vi "纳清DO电极校准.vi"() -> ()   [LabVIEW 2016, in "斯坦道多参数.lvlib"]
uses:
  <vilib>/Utility/miscctls.llb/LVPointTypeDef.ctl
  <vilib>/Analysis/NI_AALBase.lvlib
panel:
  in  "盐度自动获取":bool
  out "滤波设定":dbl
  out "标液2":string="饱和标准液"
  out "标液1":string="零点标准液"
  out "第二点信号值":dbl
  out "第一点信号值":dbl
  out "盐度":sgl format="%#.2f"
  out "大气压力":dbl format="%#.2f"
  out "饱和值":sgl format="%#.2f"
  out "报警信息":string
  out "通讯状态":string
  out "第二点校准值":dbl
  out "第一点校准值":dbl
  in  "校准停止":bool
  in  "校准启动":bool
  in  "校准模式":u16(ring)=1 items=["两点校准", "单点校准"]
  out "最小值":sgl format="%#.2f"
  out "最大值":sgl format="%#.2f"
  out "波形图表":dbl(graph) caption="历史曲线"
  out "mean":dbl caption="均值" format="%#.2f"
  out "standard deviation":dbl caption="标准差" format="%#.2f"
  out "变异系数":dbl format="%#.6f"
  out "测量值":sgl format="%#.2f"
  out "提示":string
  out "原始光强数值":sgl caption="信号值" format="%#.6f"
  out "温度":dbl format="%#.2f"
  # "DO电极设定"
  # "℃"
  # "mg/L"
  # "%"
  # "nA"
  # "kPa"
  # "ppt"
  # "请选择校准模式:"
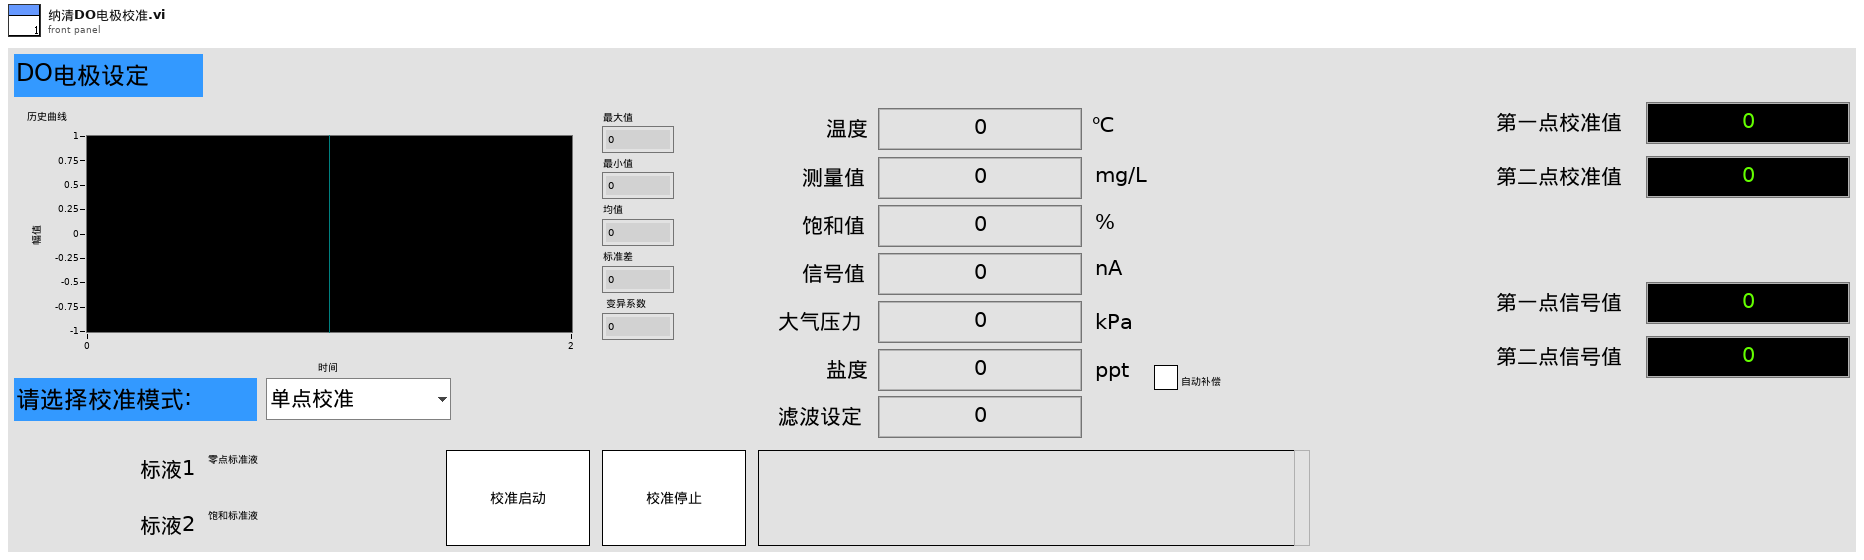
[diagram p1: front panel]
types:
  T1 = enum16{"pH", "DO", "Cond", "Turb", "ORP", "叶绿素a", "藻密度"}
  T2 = typedef "LVPointTypeDef.ctl" = cluster{"Horizontal":i16, "Vertical":i16}
  T3 = cluster{"报警码":u16, "溶解氧数值（mg/L）":sgl, "溶解氧数据（%）":sgl, "温度数据":sgl, "溶解氧原始信号 nA":sgl, "大气压力":sgl, "盐度":sgl, "0X0009_NC":string, "产品名称":string, "序列号":string, "硬件版本":string, "软件版本":string, "通讯地址":u16, "波特率":u16, "设备类型":u16, "0X0026_NC":string, "第一点原始数据":sgl, "第一点校准数据":sgl, "第二点原始数据":sgl, "第二点校准数据":sgl, "探头校准命令":u16, "温度校准参数":sgl, "温度校准命令":u16}
  T4 = cluster{"pH":u32, "DO":u32, "Cond":u32, "Turb":u32, "叶绿素a":u32, "藻密度":u32, "ORP":u32}
  T5 = enum8{"Enabled", "Disabled", "Disabled and Grayed Out"}
  T6 = cluster{"报警码":u16, "溶解氧数值（mg/L）":sgl, "溶解氧数据（%）":sgl, "温度数据":sgl, "溶解氧原始信号 nA":sgl, "大气压力":sgl, "盐度":sgl, "0X0009_NC":string, "产品名称":string, "序列号":string, "硬件版本":string, "软件版本":string, "通讯地址":u16, "波特率":u16, "设备类型":u16, "0X0026_NC":string, "第一点原始数据":sgl, "0X0033 NC":sgl, "第二点原始数据":sgl, "0X0037 NC":sgl, "探头校准命令":u16, "温度校准参数":sgl, "温度校准命令":u16}
  T7 = cluster{"ph":bool, "DO":bool, "Cond":bool, "Turb":bool, "叶绿素a":bool, "藻密度":bool, "ORP":bool}
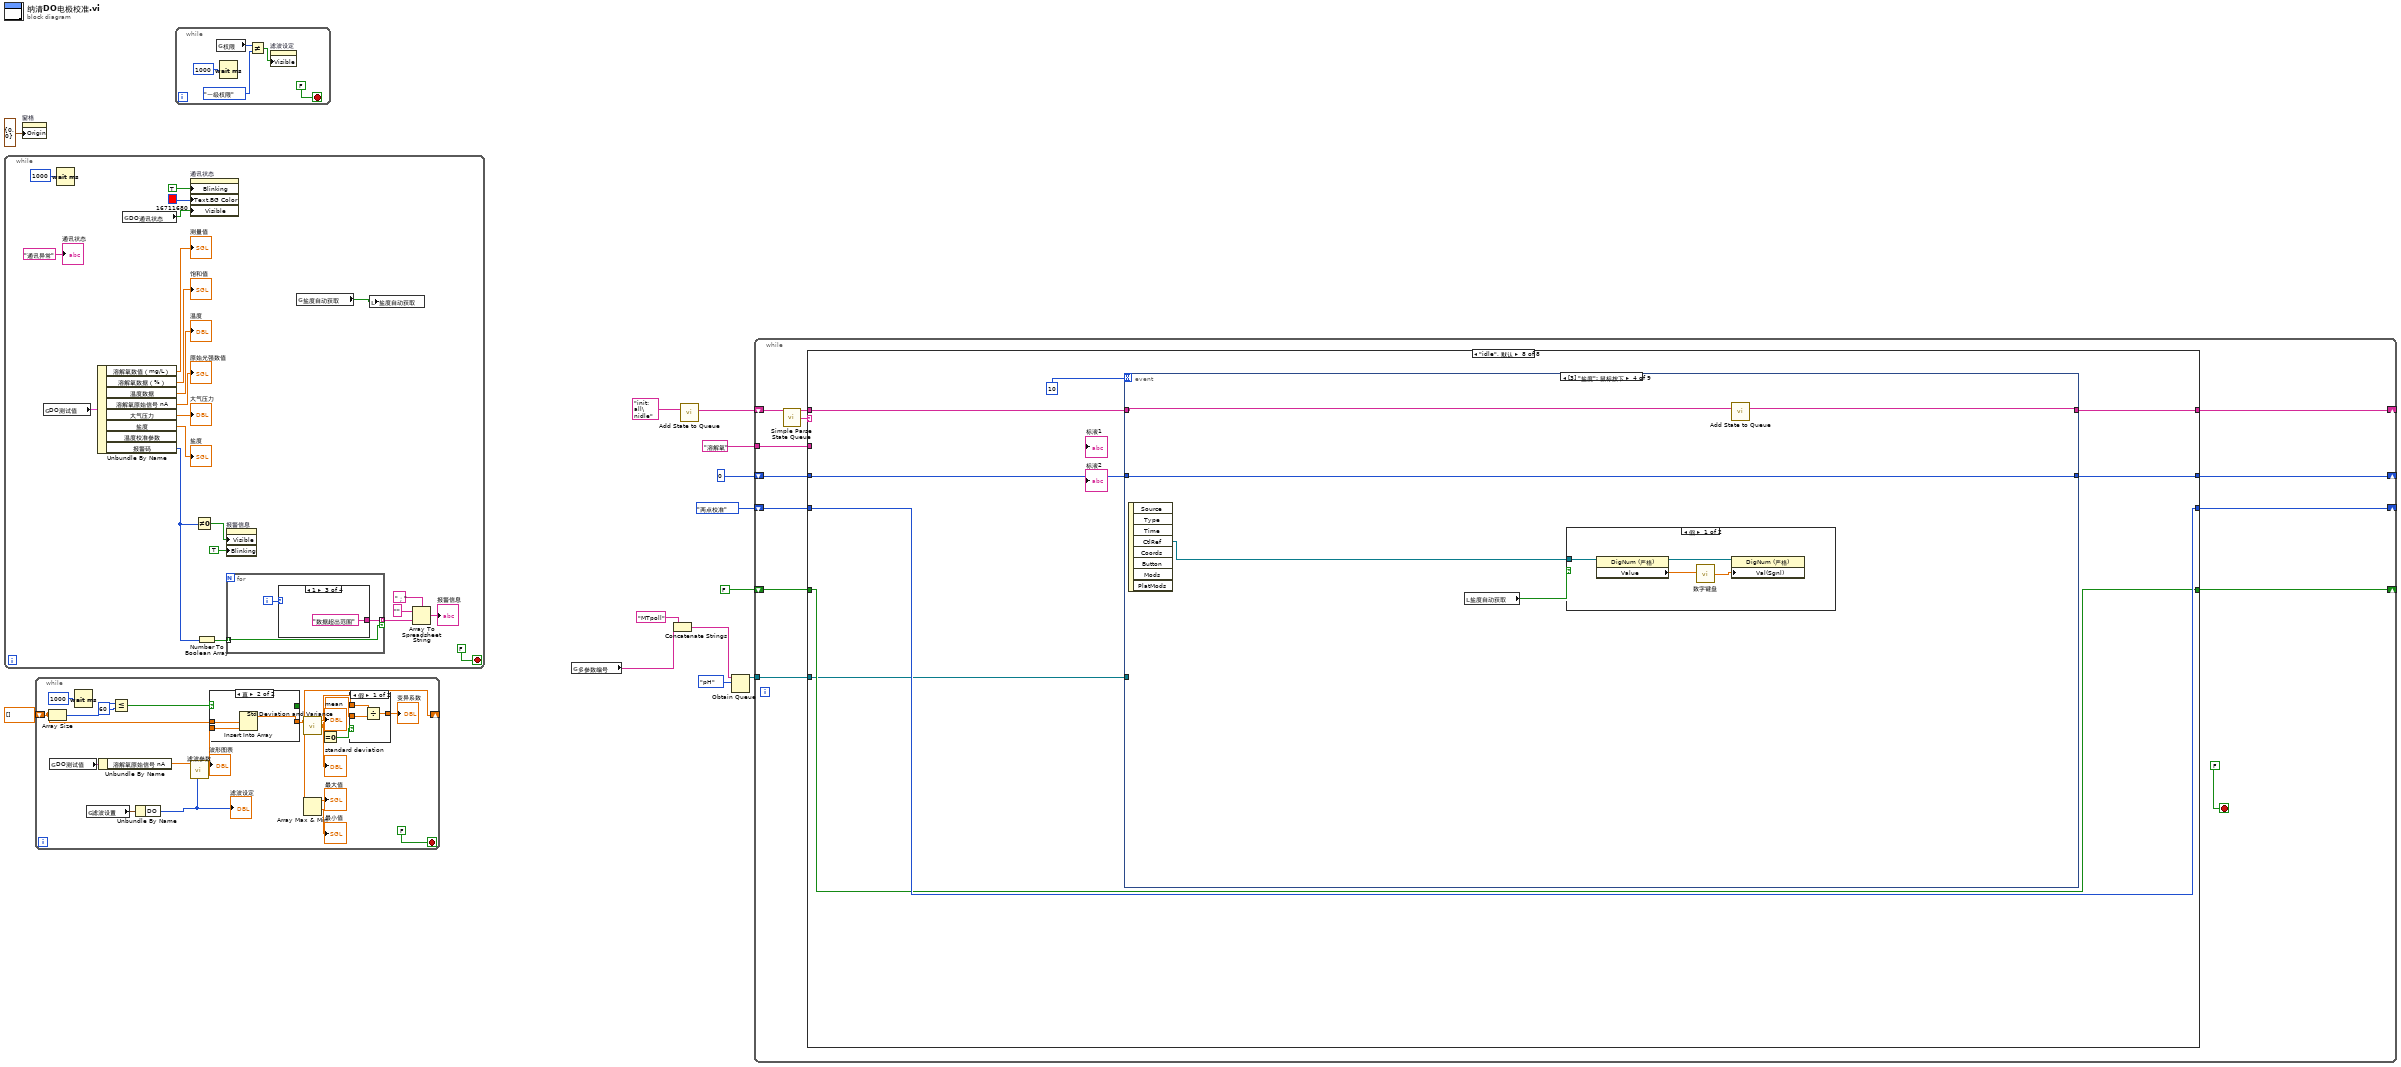
[diagram p0: block diagram]
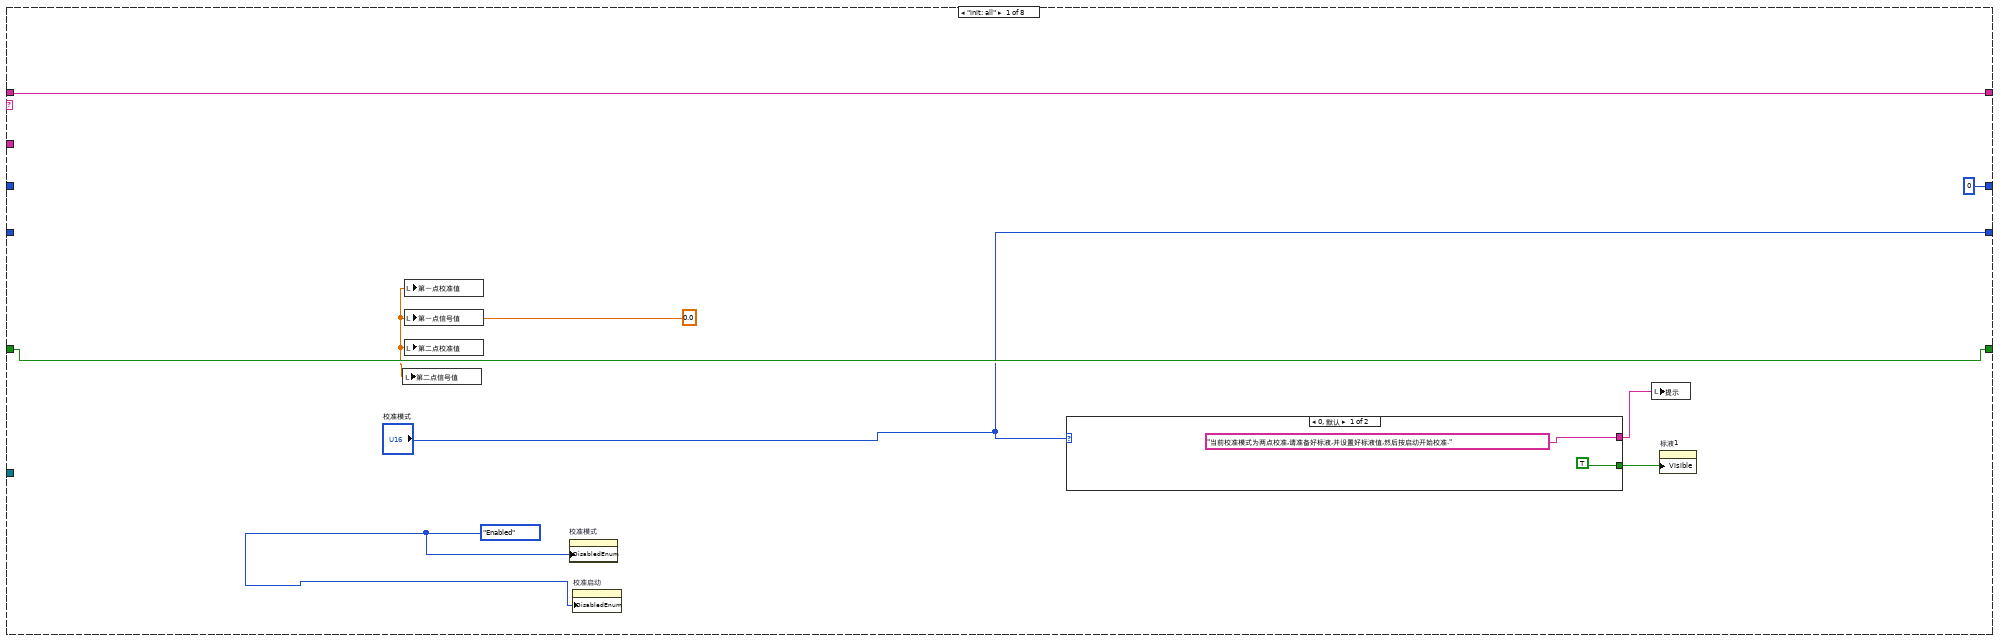
[diagram p2: hidden frame]
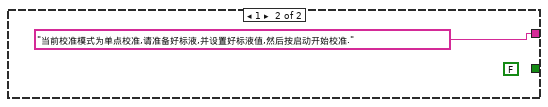
[diagram p3: hidden frame]
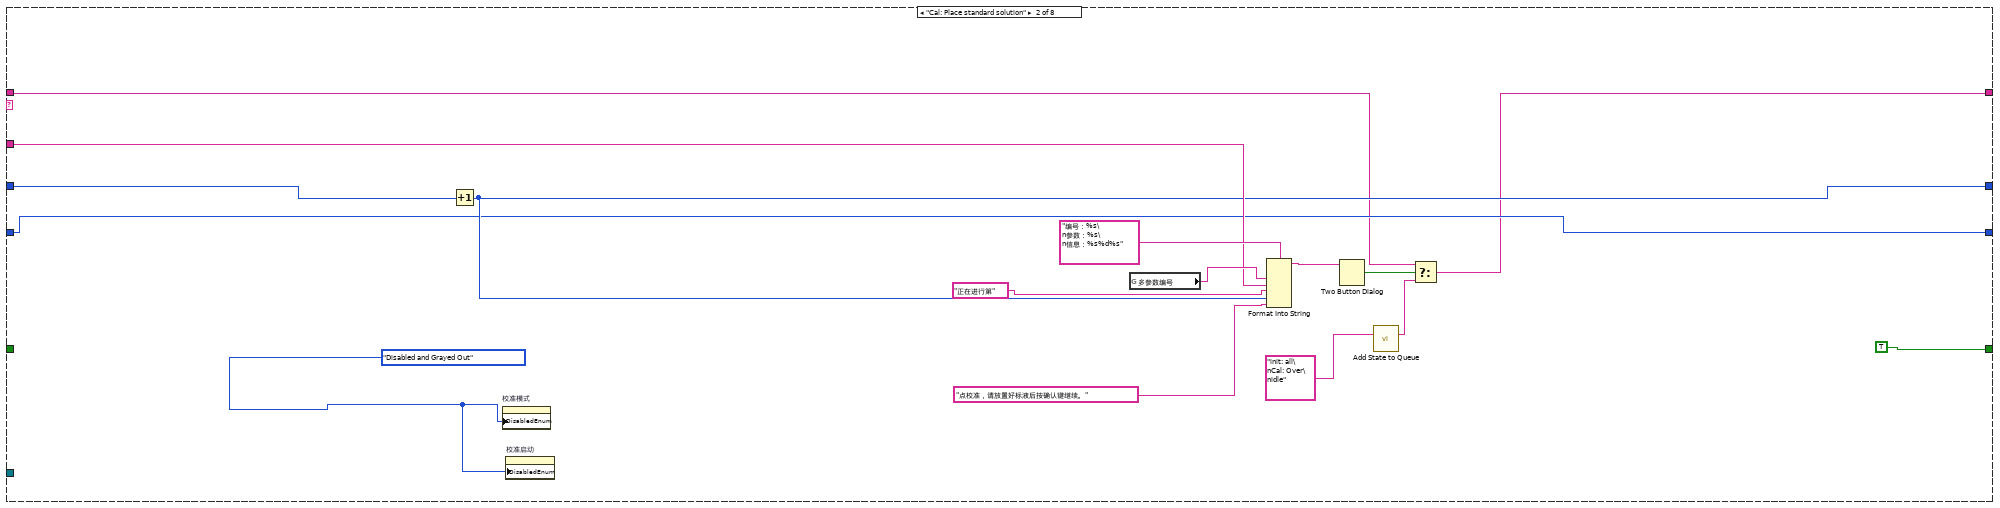
[diagram p4: hidden frame]
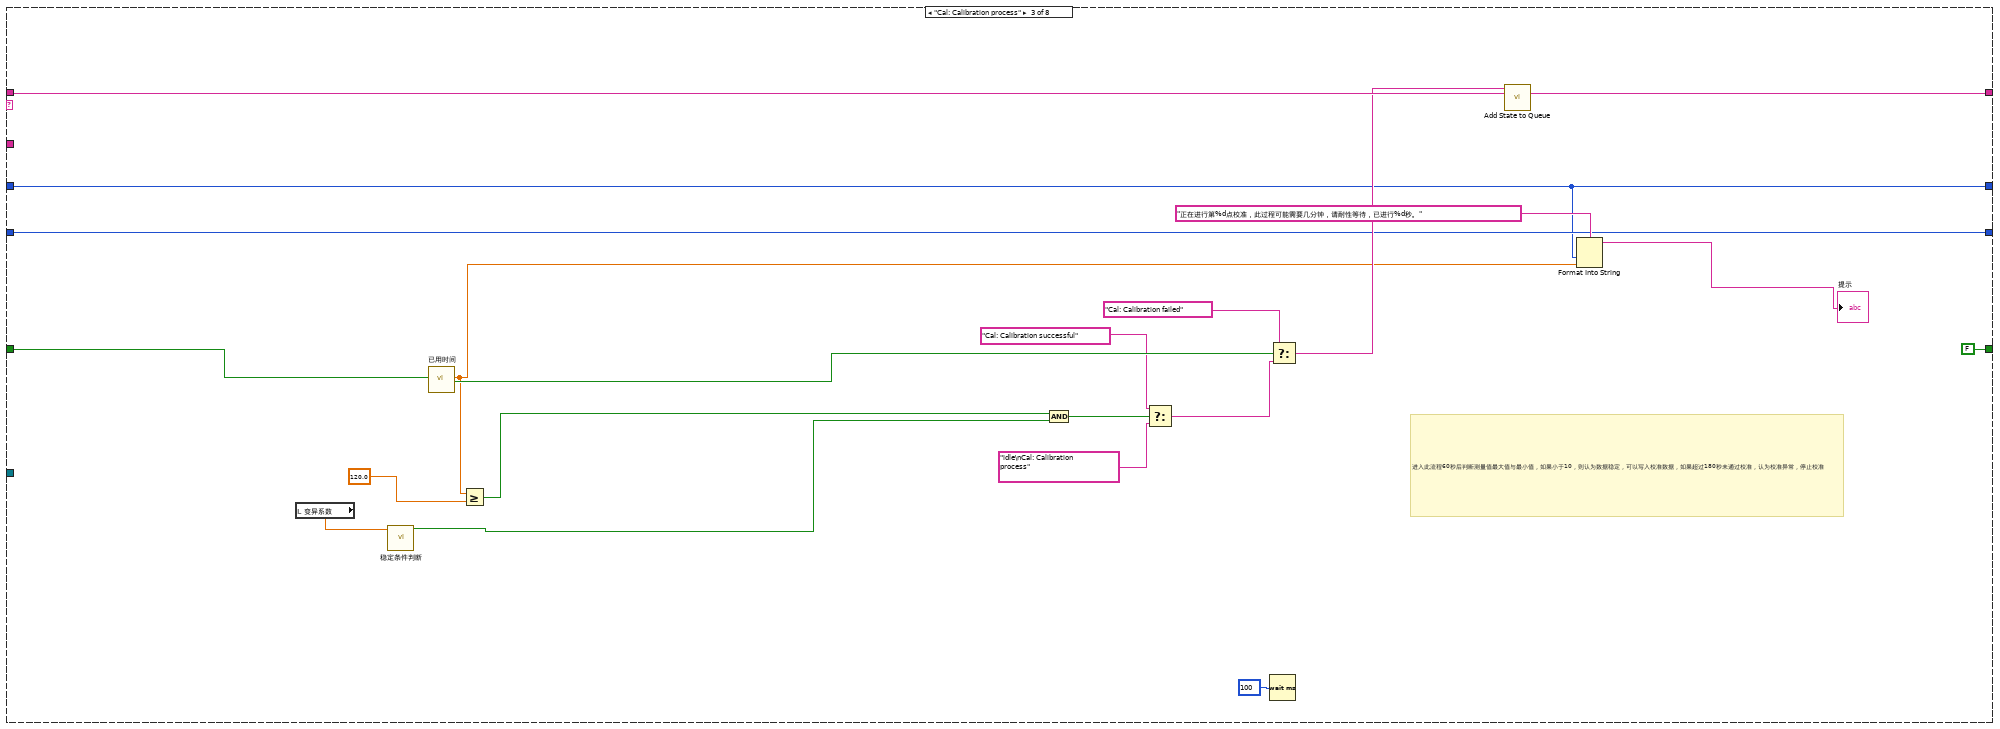
[diagram p5: hidden frame]
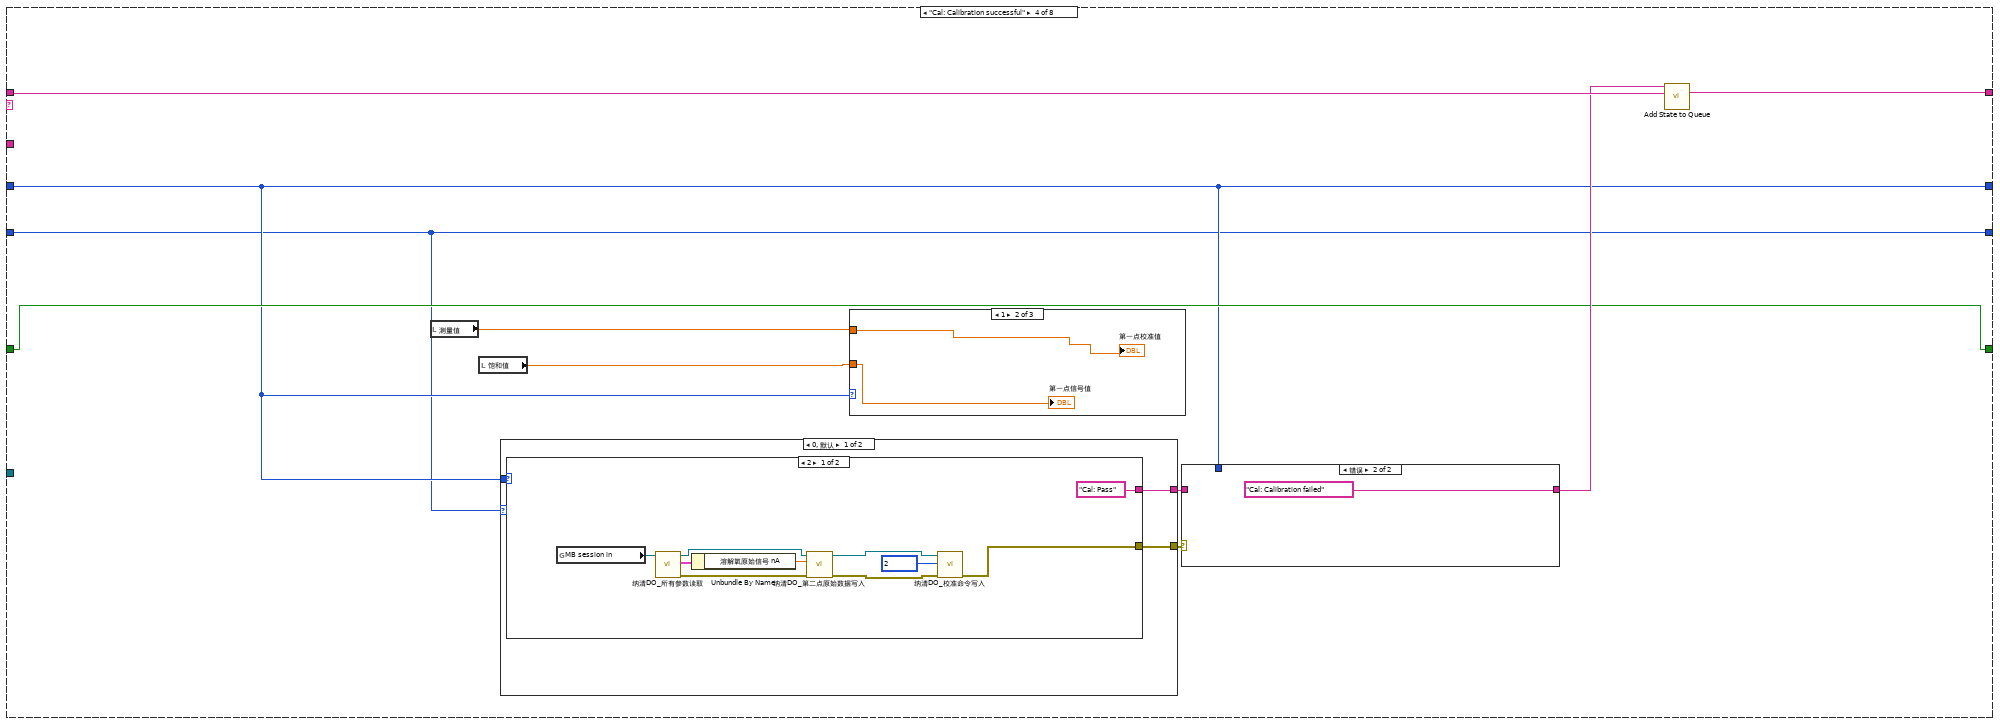
[diagram p6: hidden frame]
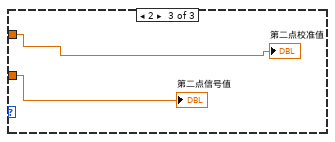
[diagram p8: hidden frame]
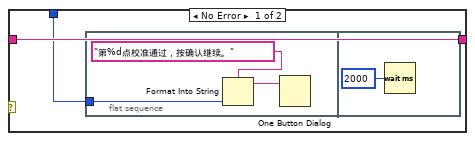
[diagram p9: hidden frame]
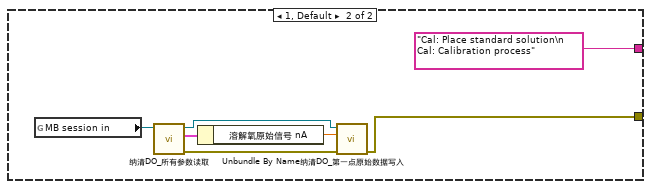
[diagram p10: hidden frame]
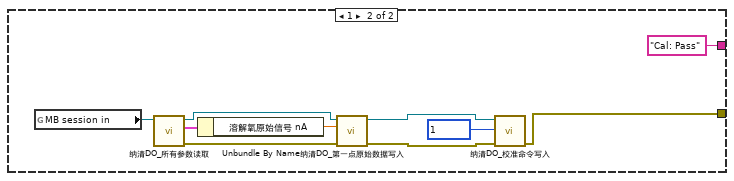
[diagram p11: hidden frame]
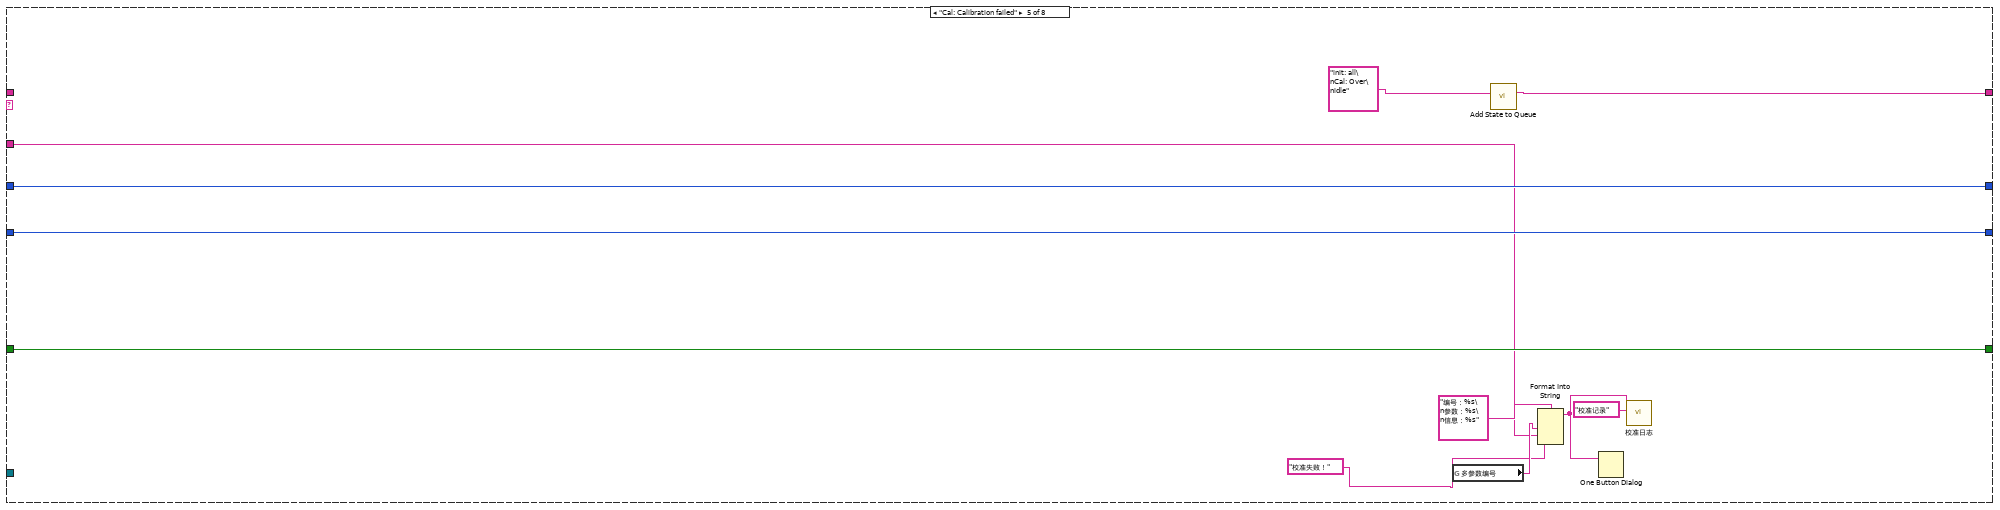
[diagram p12: hidden frame]
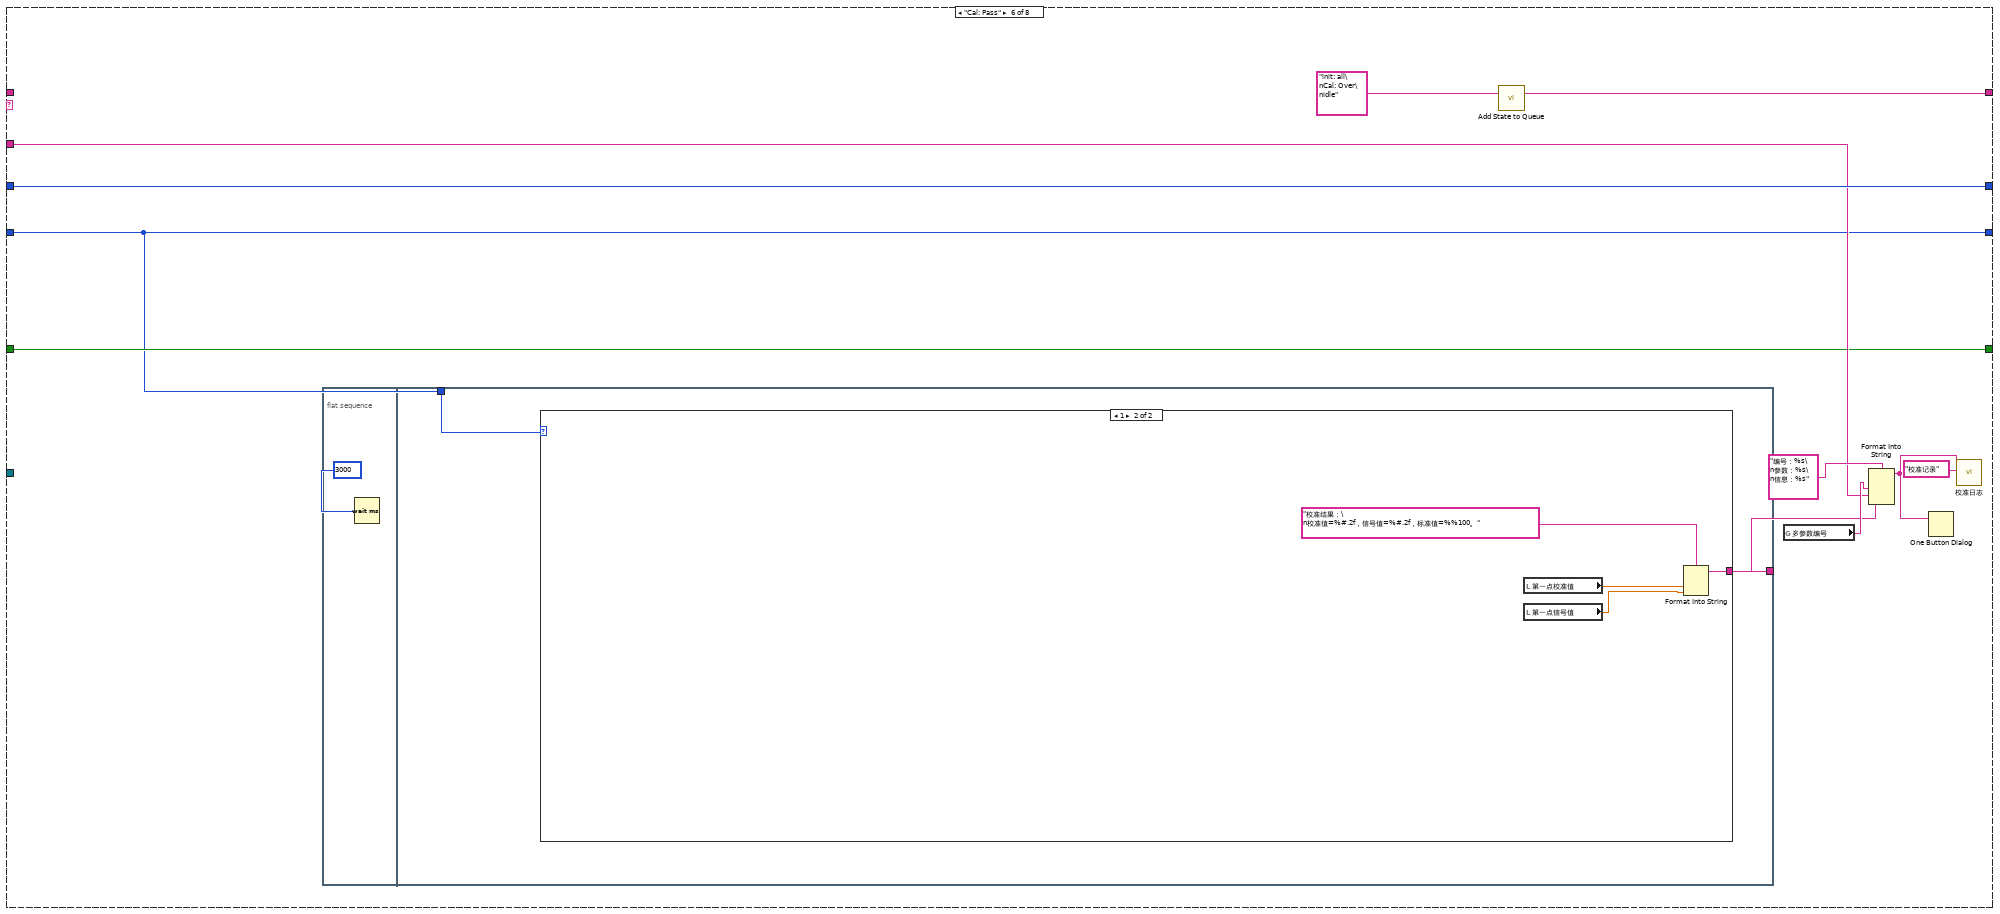
[diagram p13: hidden frame]
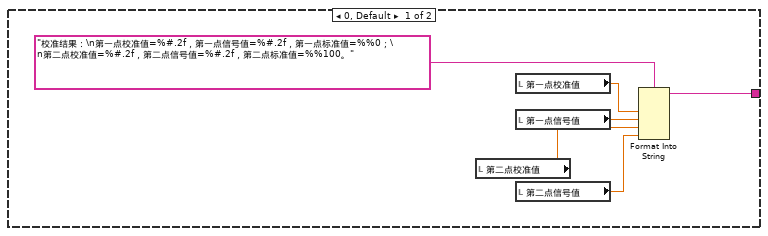
[diagram p14: hidden frame]
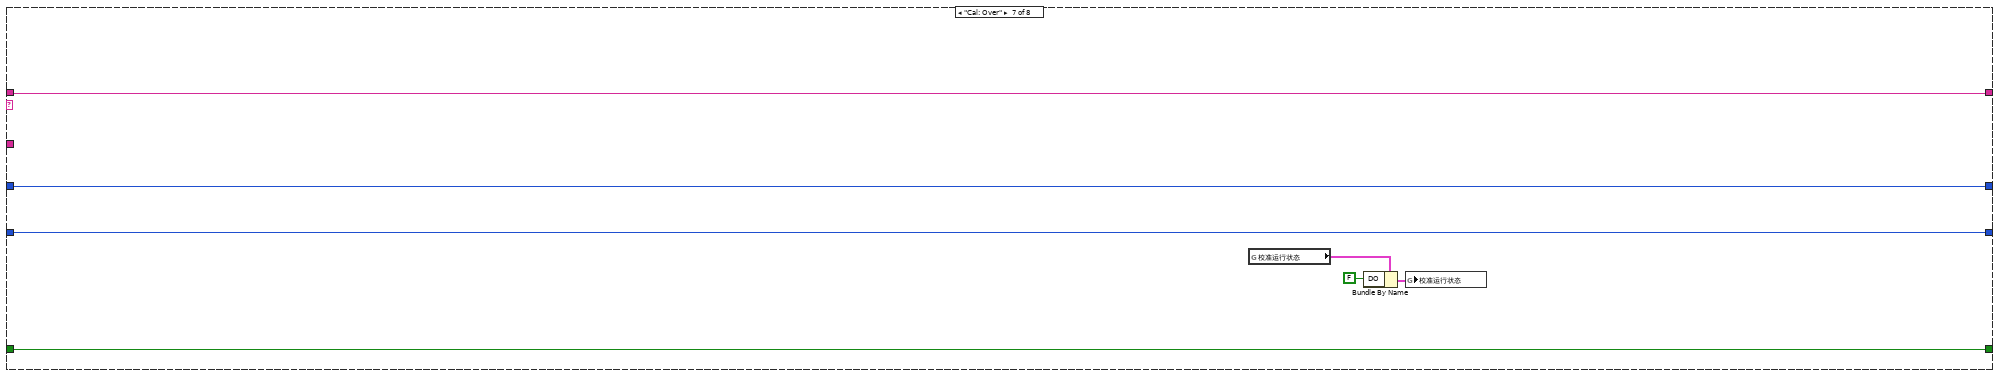
[diagram p15: hidden frame]
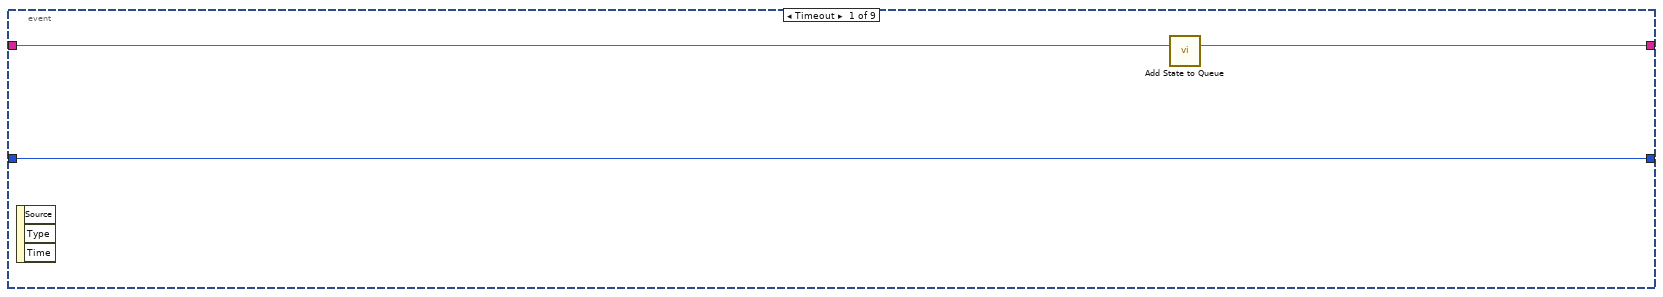
[diagram p16: hidden frame]
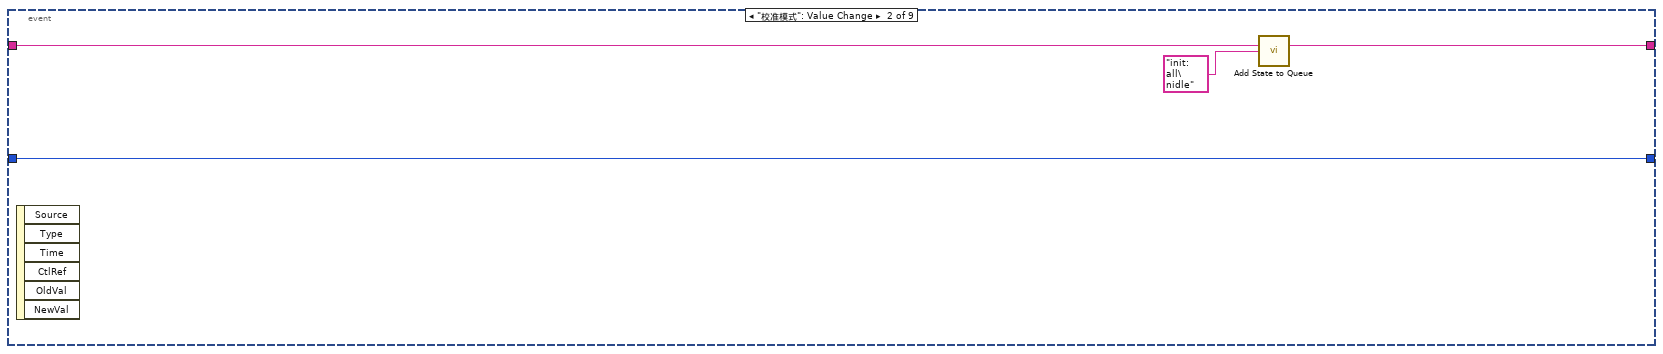
[diagram p17: hidden frame]
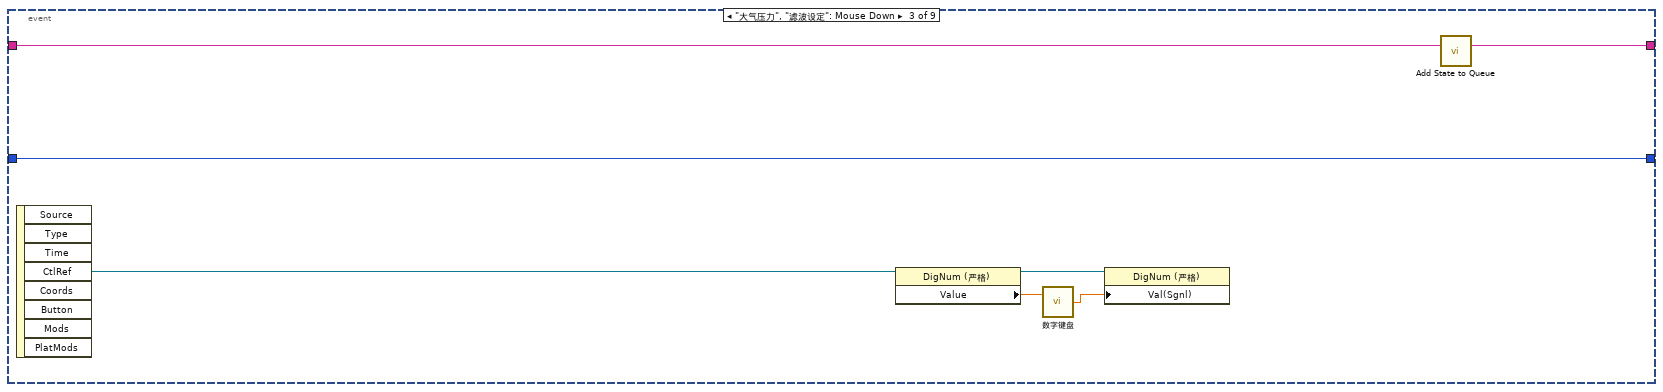
[diagram p18: hidden frame]
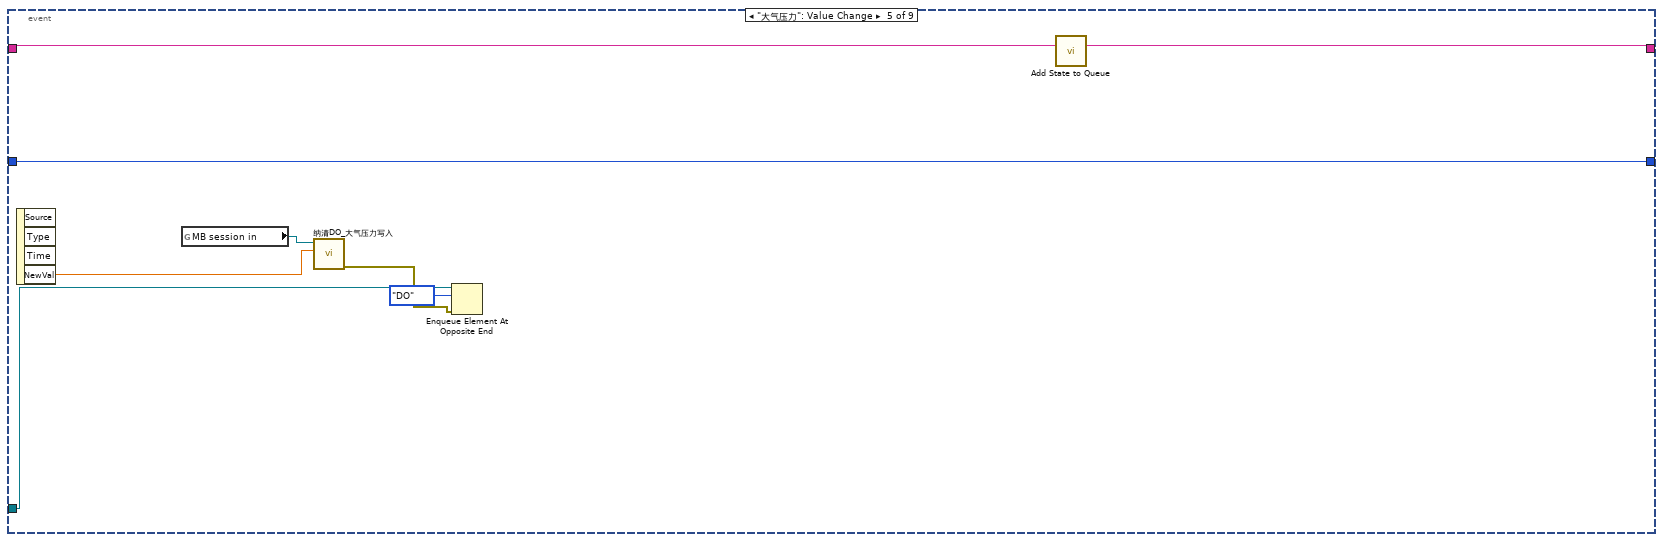
[diagram p20: hidden frame]
diagram:
  n1 = while {
    stop <- FALSE stop-if-true
    n2 = global read "纳清过程全局变量.vi" "DO测试值"() -> (w33:T3)
    n3 = Wait (ms)(milliseconds to wait=u32 1000 ("等待时间（毫秒）")) -> ()  [unwired: 1 out]
    n4 = Unbundle By Name(w33) -> ("溶解氧数值（mg/L）"=→"测量值":sgl, "溶解氧数据（%）"=→"饱和值":sgl, "温度数据"=→"温度":sgl, "溶解氧原始信号 nA"=→"原始光强数值":sgl, "大气压力"=→"大气压力":sgl, "盐度"=→"盐度":sgl, "报警码"=w20:u16)  [unwired: 1 out]
    n5 = global read "多参数全局变量.vi" "DO通讯状态"() -> (w26:bool)
    n6 = property on="通讯状态" class="Str"("Blinking"=TRUE ("闪烁"), "Text.BG Color"=u32 16711680, "Visible"=w26) -> ()  [unwired: 2 in, 2 out]
    n7 = Not Equal To 0?(x=w20) -> (x != 0?=w19:bool)
    n8 = Number To Boolean Array(number=w20) -> (Boolean array=w25:bool[])
    n9 = property on="报警信息" class="Str"("Visible"=w19, "Blinking"=TRUE ("闪烁")) -> ()  [unwired: 2 in, 2 out]
    n10 = for {
      tunnel: w25 -> [w36] mode=indexing
      tunnel: [w37] -> w24 mode=indexing if=w36
      i -> [w38]
      n11 = case shown="1" w38 {
        tunnel: [_ "温度超出范围" "数据超出范围" "温度传感器故障"] -> w37
        frame Default {
        }
        frame 0 {
        }
        frame 1 {
        }
        frame 8 {
        }
      }
    }
    n12 = global read "断电保存变量.vi" "盐度自动获取"() -> (w14:bool)
    n13 = local write "盐度自动获取"(w14) -> ()
    n14 = Array To Spreadsheet String(delimiter (Tab)="；" ("分隔符(Tab)"), array=w24, 3:"" ("格式字符串")) -> (spreadsheet string=→"报警信息":string)
    "通讯状态" <- "通讯异常" ("当前串口")
  }
  n15 = property on="窗格" class="Pane"("Origin"=T2 {"Horizontal"=0, "Vertical"=0} ("原点")) -> ()  [unwired: 2 in, 2 out]
  n16 = while {
    shift-right: [w49] -> _
    shift-left: sgl[] [] -> [w55]
    stop <- FALSE stop-if-true
    n17 = Array Size(array=w55) -> (size(s)=w57:i32)
    n18 = global read "纳清过程全局变量.vi" "DO测试值"() -> (w46:T3)
    n19 = Wait (ms)(milliseconds to wait=u32 1000 ("等待时间（毫秒）")) -> ()  [unwired: 1 out]
    n20 = global read "断电保存变量.vi" "滤波设置"() -> (w43:T4)
    n21 = Unbundle By Name(w46) -> ("溶解氧原始信号 nA"=w45:sgl)
    n22 = Less Or Equal?(x=w57, y=60) -> (x <= y?=w56:bool)
    n23 = Unbundle By Name(w43) -> ("DO"=w42:u32)
    "滤波设定" <- w42
    n24 = call "滤波参数.vi"("滤波次数"=w42, "x"=w45) -> ("mode"=w44:dbl)  [unwired: 9 in]
    "波形图表" <- w44
    n25 = case shown="真" w56 {
      tunnel: w55 -> [w68 w71]
      tunnel: w44 -> [w66 w70]
      tunnel: [w64 w69] -> w49
      tunnel: [TRUE _] -> _
      frame False {
        n26 = Replace Array Subset(array=w68, new element=w66) -> (w67:sgl[])  [unwired: 1 in]
        n27 = Rotate 1D Array(1:w67, 2:-1 ("n")) -> (0:w64:sgl[])
      }
      frame True {
        n28 = Insert Into Array(array=w71, new element=w70) -> (w69:sgl[])  [unwired: 1 in]
      }
    }
    n29 = call <vilib>:"Std Deviation and Variance.vi"("X"=w49) -> ("mean"=w53:dbl, "standard deviation"=w52:dbl)  [unwired: 1 in, 1 out]
    "mean" <- w53
    "standard deviation" <- w52
    n30 = Array Max & Min(array=w49) -> (max value=→"最大值":sgl, min value=→"最小值":sgl)  [unwired: 2 out]
    n31 = Equal To 0?(x=w53) -> (x = 0?=w54:bool)
    n32 = case shown="假" w54 {
      tunnel: w52 -> [w62 _]
      tunnel: [w61 _] -> w51
      tunnel: w53 -> [w60 _]
      frame False {
        n33 = Divide(x=w62, y=w60) -> (x/y=w61:dbl)
      }
      frame True {
      }
    }
    "变异系数" <- w51
  }
  n34 = while {
    stop <- FALSE stop-if-true
    n35 = global read "多参数全局变量.vi" "权限"() -> (w75:enum16{"一级权限", "二级权限", "三级权限"})
    n36 = Wait (ms)(milliseconds to wait=u32 1000 ("等待时间（毫秒）")) -> ()  [unwired: 1 out]
    n37 = Not Equal?(x=w75, y=enum16{"一级权限", "二级权限", "三级权限"}."一级权限") -> (x != y?=w72:bool)
    n38 = property on="滤波设定" class="DigNum (严格)"("Visible"=w72) -> ()  [unwired: 2 in, 2 out]
  }
  n39 = global read "多参数全局变量.vi" "多参数编号"() -> (w2:string)
  n40 = Concatenate Strings("MTpoll" ("名称（未命名）"), w2) -> (w4:string)
  n41 = call "Add State to Queue.vi"("State(s) In (\"\")"="init: all\nidle" ("State(s) In (\"\")")) -> ("States Out"=w10:string)  [unwired: 14 in]
  n42 = Obtain Queue(name (unnamed)=w4, element data type=T1."pH" ("枚举")) -> (queue out=w1:refnum<queue>)  [unwired: 3 in, 2 out]
  n43 = while {
    shift-right: [w85] -> _
    shift-left: w10 -> [w89]
    shift-right: [w82] -> _
    shift-left: 0 -> [w84]
    tunnel: "溶解氧" ("State(s) In (\"\")") -> [w83]
    shift-right: [w80] -> _
    shift-left: enum16{"两点校准", "单点校准"}."两点校准" ("校准模式") -> [w81]
    shift-right: [w78] -> _
    shift-left: FALSE -> [w79]
    tunnel: w1 -> [w77]
    stop <- FALSE stop-if-true
    n44 = call "Simple Parse State Queue.vi"("State Queue"=w89) -> ("Remain States"=w86:string, "Next State"=w87:string)  [unwired: 13 in]
    n45 = case shown="\"idle\", 默认" w87 {
      tunnel: w86 -> [w97 w104 w136 w145 _ _ w230 w238]
      tunnel: [w97 w103 w135 w144 w196 w201 w230 w237] -> w85
      tunnel: w84 -> [_ w112 w121 w139 w199 w210 w229 w235]
      tunnel: w83 -> [_ w113 _ _ w190 w206 _ _]
      tunnel: [0 w110 w121 w139 w199 w210 w229 w236] -> w82
      tunnel: w81 -> [_ w109 w122 w138 w198 w202 w228 w234]
      tunnel: ["校准模式" w109 w122 w138 w198 w202 w228 w234] -> w80
      tunnel: w79 -> [w94 _ w124 w140 w197 w205 w227 w232]
      tunnel: [w94 TRUE FALSE w140 w197 w205 w227 w232] -> w78
      tunnel: w77 -> [_ _ _ _ _ _ _ w231]
      frame "init: all" {
        w91 = T5."Enabled" ("禁用")
        w93 = 0.0 ("第一点校准值")
        n46 = local write "第二点信号值"(w93) -> ()
        n47 = local write "第一点校准值"(w93) -> ()
        n48 = local write "第一点信号值"(w93) -> ()
        n49 = local write "第二点校准值"(w93) -> ()
        n50 = property on="校准模式" class="Ring (严格)"("DisabledEnum"=w91) -> ()  [unwired: 2 in, 2 out]
        n51 = property on="校准启动" class="Bool"("DisabledEnum"=w91) -> ()  [unwired: 2 in, 2 out]
        n52 = case shown="0, 默认" "校准模式" {
          tunnel: ["当前校准模式为两点校准,请准备好标液,并设置好标液值,然后按启动开始校准." ("提示") "当前校准模式为单点校准,请准备好标液,并设置好标液值,然后按启动开始校准." ("提示")] -> w96
          tunnel: [TRUE ("可见") _] -> w90
          frame 0, Default {
          }
          frame 1 {
            (unwired) FALSE ("可见")
          }
        }
        n53 = local write "提示"(w96) -> ()
        n54 = property on="标液1" class="Str"("Visible"=w90) -> ()  [unwired: 2 in, 2 out]
      }
      frame "Cal: Place standard solution" {
        w102 = T5."Disabled and Grayed Out" ("禁用")
        n55 = Increment(x=w112) -> (x+1=w110:i32)
        n56 = property on="校准模式" class="Ring (严格)"("DisabledEnum"=w102) -> ()  [unwired: 2 in, 2 out]
        n57 = property on="校准启动" class="Bool"("DisabledEnum"=w102) -> ()  [unwired: 2 in, 2 out]
        n58 = global read "多参数全局变量.vi" "多参数编号"() -> (w115:string)
        n59 = Format Into String(format string="编号：%s\n参数：%s\n信息：%s%d%s" ("格式字符串"), w115, w113, "正在进行第" ("消息"), w110, "点校准，请放置好标液后按确认键继续。" ("消息")) -> (resulting string=w107:string)  [unwired: 2 in, 1 out]
        n60 = Two Button Dialog(message=w107) -> (T button?=w106:bool)  [unwired: 2 in]
        n61 = call "Add State to Queue.vi"("State(s) In (\"\")"="init: all\nCal: Over\nidle" ("State(s) In (\"\")")) -> ("States Out"=w105:string)  [unwired: 14 in]
        n62 = Select(t=w104, s=w106, f=w105) -> (s? t:f=w103:string)
      }
      frame "Cal: Calibration process" {
        # "进入此流程60秒后判断测量值最大值与最小值，如果小于10，则认为数据稳定，可以写入校准数据，如果超过180秒未通过校准，认为校准异常，停止校准"
        n63 = local read "变异系数"() -> (w118:dbl)
        n64 = call "稳定条件判断.vi"("变异系数"=w118) -> ("布尔"=w117:bool)  [unwired: 10 in]
        n65 = call "已用时间"("Reset"=w124) -> ("Elapsed Time (s)"=w120:dbl, "Time has Elapsed"=w137:bool)  [unwired: 11 in, 6 out]
        n66 = Greater Or Equal?(x=w120, y=120.0) -> (x >= y?=w132:bool)
        n67 = And(x=w132, y=w117) -> (x .and. y?=w129:bool)
        n68 = Select(t="Cal: Calibration successful" ("State(s) In (\"\")"), s=w129, f="idle\nCal: Calibration process" ("State(s) In (\"\")")) -> (s? t:f=w128:string)
        n69 = Wait (ms)(milliseconds to wait=u32 100 ("等待时间（毫秒）")) -> ()  [unwired: 1 out]
        n70 = Select(t="Cal: Calibration failed" ("State(s) In (\"\")"), s=w137, f=w128) -> (s? t:f=w127:string)
        n71 = call "Add State to Queue.vi"("State(s) In Front (\"\")"=w127, "State(s) In (\"\")"=w136) -> ("States Out"=w135:string)  [unwired: 13 in]
        n72 = Format Into String(format string="正在进行第%d点校准，此过程可能需要几分钟，请耐性等待，已进行%d秒。" ("格式字符串"), w121, w120) -> (resulting string=→"提示":string)  [unwired: 2 in, 1 out]
      }
      frame "Cal: Calibration successful" {
        n73 = local read "测量值"() -> (w141:sgl)
        n74 = local read "饱和值"() -> (w142:sgl)
        n75 = case shown="0, 默认" w138 {
          tunnel: [w161 w179] -> w147
          tunnel: [w160 "Cal: Pass" ("State(s) In (\"\")")] -> w146
          tunnel: w139 -> [w159 _]
          frame 0, Default {
            n76 = case shown="2" w159 {
              tunnel: [w163 w172] -> w161
              tunnel: ["Cal: Pass" ("State(s) In (\"\")") "Cal: Place standard solution\n Cal: Calibration process" ("State(s) In (\"\")")] -> w160
              frame 2 {
                n77 = global read "多参数全局变量.vi" "MB session in"() -> (w168:refnum<class "MB_Master.lvclass">)
                n78 = call "纳清DO_所有参数读取.vi"("MB session in"=w168) -> ("error out"=w170:errorcluster, "输出值"=w167:T6, "MB session out"=w169:refnum<class "MB_Master.lvclass">)  [unwired: 8 in]
                n79 = Unbundle By Name(w167) -> ("溶解氧原始信号 nA"=w166:sgl)
                n80 = call "纳清DO_第二点原始数据写入.vi"("error in (no error)"=w170, "数值"=w166, "MB session in"=w169) -> ("error out"=w165:errorcluster, "MB session out"=w164:refnum<class "MB_Master.lvclass">)  [unwired: 7 in]
                n81 = call "纳清DO_校准命令写入.vi"("error in (no error)"=w165, "数值"=u16 2 ("starting address"), "MB session in"=w164) -> ("error out"=w163:errorcluster)  [unwired: 7 in, 1 out]
              }
              frame 1, Default {
                n82 = global read "多参数全局变量.vi" "MB session in"() -> (w175:refnum<class "MB_Master.lvclass">)
                n83 = call "纳清DO_所有参数读取.vi"("MB session in"=w175) -> ("error out"=w177:errorcluster, "输出值"=w174:T6, "MB session out"=w176:refnum<class "MB_Master.lvclass">)  [unwired: 8 in]
                n84 = Unbundle By Name(w174) -> ("溶解氧原始信号 nA"=w173:sgl)
                n85 = call "纳清DO_第一点原始数据写入.vi"("error in (no error)"=w177, "数值"=w173, "MB session in"=w176) -> ("error out"=w172:errorcluster)  [unwired: 7 in, 1 out]
              }
            }
          }
          frame 1 {
            n86 = global read "多参数全局变量.vi" "MB session in"() -> (w185:refnum<class "MB_Master.lvclass">)
            n87 = call "纳清DO_所有参数读取.vi"("MB session in"=w185) -> ("error out"=w187:errorcluster, "输出值"=w184:T6, "MB session out"=w186:refnum<class "MB_Master.lvclass">)  [unwired: 8 in]
            n88 = Unbundle By Name(w184) -> ("溶解氧原始信号 nA"=w183:sgl)
            n89 = call "纳清DO_第一点原始数据写入.vi"("error in (no error)"=w187, "数值"=w183, "MB session in"=w186) -> ("error out"=w182:errorcluster, "MB session out"=w181:refnum<class "MB_Master.lvclass">)  [unwired: 7 in]
            n90 = call "纳清DO_校准命令写入.vi"("error in (no error)"=w182, "数值"=u16 1 ("starting address"), "MB session in"=w181) -> ("error out"=w179:errorcluster)  [unwired: 7 in, 1 out]
          }
        }
        n91 = case shown="1" w139 {
          tunnel: w142 -> [_ w149 w151]
          tunnel: w141 -> [_ w148 w150]
          frame 0, Default {
          }
          frame 1 {
            "第一点信号值" <- w149
            "第一点校准值" <- w148
          }
          frame 2 {
            "第二点信号值" <- w151
            "第二点校准值" <- w150
          }
        }
        n92 = case shown="错误" w147 {
          tunnel: w146 -> [w153 _]
          tunnel: [w153 "Cal: Calibration failed" ("State(s) In (\"\")")] -> w143
          tunnel: w139 -> [w152 _]
          frame No Error {
            n93 = flat-sequence {
              tunnel: w152 -> [w154]
              frame #0 {
                n94 = Format Into String(format string="第%d点校准通过，按确认继续。" ("格式字符串"), w154) -> (resulting string=w156:string)  [unwired: 2 in, 1 out]
                n95 = One Button Dialog(message=w156) -> ()  [unwired: 1 in, 1 out]
              }
              frame #1 {
                n96 = Wait (ms)(milliseconds to wait=u32 2000 ("等待时间（毫秒）")) -> ()  [unwired: 1 out]
              }
            }
          }
          frame Error {
          }
        }
        n97 = call "Add State to Queue.vi"("State(s) In Front (\"\")"=w143, "State(s) In (\"\")"=w145) -> ("States Out"=w144:string)  [unwired: 13 in]
      }
      frame "Cal: Calibration failed" {
        n98 = global read "多参数全局变量.vi" "多参数编号"() -> (w193:string)
        n99 = call "Add State to Queue.vi"("State(s) In (\"\")"="init: all\nCal: Over\nidle" ("State(s) In (\"\")")) -> ("States Out"=w196:string)  [unwired: 14 in]
        n100 = Format Into String(format string="编号：%s\n参数：%s\n信息：%s" ("格式字符串"), w193, w190, "校准失败！" ("消息")) -> (resulting string=w192:string)  [unwired: 2 in, 1 out]
        n101 = One Button Dialog(message=w192) -> ()  [unwired: 1 in, 1 out]
        n102 = call "校准日志.vi"("table"="校准记录", "日志信息"=w192) -> ()  [unwired: 9 in, 1 out]
      }
      frame "Cal: Pass" {
        n103 = flat-sequence {
          tunnel: [w213] -> w203
          tunnel: w202 -> [w212]
          frame #0 {
            n104 = Wait (ms)(milliseconds to wait=u32 3000 ("等待时间（毫秒）")) -> ()  [unwired: 1 out]
          }
          frame #1 {
            n105 = case shown="1" w212 {
              tunnel: [w219 w223] -> w213
              frame 0, Default {
                n106 = local read "第二点校准值"() -> (w215:dbl)
                n107 = local read "第一点校准值"() -> (w217:dbl)
                n108 = local read "第一点信号值"() -> (w218:dbl)
                n109 = local read "第二点信号值"() -> (w214:dbl)
                n110 = Format Into String(format string="校准结果：\n第一点校准值=%#.2f，第一点信号值=%#.2f，第一点标准值=%%0；\n第二点校准值=%#.2f，第二点信号值=%#.2f，第二点标准值=%%100。" ("提示"), w217, w218, w215, w214) -> (resulting string=w219:string)  [unwired: 2 in, 1 out]
              }
              frame 1 {
                n111 = local read "第一点校准值"() -> (w222:dbl)
                n112 = local read "第一点信号值"() -> (w220:dbl)
                n113 = Format Into String(format string="校准结果：\n校准值=%#.2f，信号值=%#.2f，标准值=%%100。" ("提示"), w222, w220) -> (resulting string=w223:string)  [unwired: 2 in, 1 out]
              }
            }
          }
        }
        n114 = call "Add State to Queue.vi"("State(s) In (\"\")"="init: all\nCal: Over\nidle" ("State(s) In (\"\")")) -> ("States Out"=w201:string)  [unwired: 14 in]
        n115 = global read "多参数全局变量.vi" "多参数编号"() -> (w207:string)
        n116 = Format Into String(format string="编号：%s\n参数：%s\n信息：%s" ("格式字符串"), w207, w206, w203) -> (resulting string=w204:string)  [unwired: 2 in, 1 out]
        n117 = One Button Dialog(message=w204) -> ()  [unwired: 1 in, 1 out]
        n118 = call "校准日志.vi"("table"="校准记录", "日志信息"=w204) -> ()  [unwired: 9 in, 1 out]
      }
      frame "Cal: Over" {
        n119 = global read "多参数全局变量.vi" "校准运行状态"() -> (w225:T7)
        n120 = Bundle By Name(cluster=w225, "DO"=FALSE) -> (w226:T7)
        n121 = global write "多参数全局变量.vi" "校准运行状态"(w226) -> ()
      }
      frame "idle", Default {
        n122 = event shown="[3] \"盐度\": 鼠标按下" {
          selector: _ -> [_ _ _ _ _ _ _ _ _]
          dyn-events: _ -> [_ _ _ _ _ _ _ _ _]
          timeout: 10 -> [_ _ _ _ _ _ _ _ _]
          tunnel: w238 -> [w241 w245 w250 w254 w265 w270 w282 _ w288]
          tunnel: [w240 w244 w251 w257 w269 w272 w281 w284 w287] -> w237
          tunnel: [w239 w242 w252 w256 w268 w271 w279 w285 w286] -> w236
          tunnel: w235 -> [w239 w242 w252 w256 w268 w271 w279 w285 w286]
          tunnel: w231 -> [_ _ _ _ w263 _ _ _ _]
          event Timeout {
            n123 = event-data() -> ()  [unwired: 1 in, 3 out]
            n124 = call "Add State to Queue.vi"("State(s) In (\"\")"=w241) -> ("States Out"=w240:string)  [unwired: 14 in]
          }
          event "校准模式": Value Change {
            n125 = event-data() -> ()  [unwired: 1 in, 6 out]
            n126 = call "Add State to Queue.vi"("State(s) In (\"\")"=w245, "State(s) At Back (\"\")"="init: all\nidle" ("State(s) In (\"\")")) -> ("States Out"=w244:string)  [unwired: 13 in]
          }
          event "大气压力", "滤波设定": Mouse Down {
            n127 = event-data() -> ("CtlRef"=w249:refnum<vi>)  [unwired: 1 in, 7 out]
            n128 = property class="DigNum (严格)"(reference=w249) -> (reference out=w246:refnum<vi>, "Value"=w247:dbl)  [unwired: 1 in, 1 out]
            n129 = call "数字键盘.vi"("OldNumber"=w247) -> ("NewNumber"=w248:dbl)  [unwired: 1 in]
            n130 = property class="DigNum (严格)"(reference=w246, "Val(Sgnl)"=w248) -> ()  [unwired: 1 in, 2 out]
            n131 = call "Add State to Queue.vi"("State(s) In (\"\")"=w250) -> ("States Out"=w251:string)  [unwired: 14 in]
          }
          event "盐度": Mouse Down {
            n132 = event-data() -> ("CtlRef"=w255:refnum<vi>)  [unwired: 1 in, 7 out]
            n133 = local read "盐度自动获取"() -> (w253:bool)
            n134 = case shown="假" w253 {
              tunnel: w255 -> [w261 _]
              frame False {
                n135 = property class="DigNum (严格)"(reference=w261) -> (reference out=w259:refnum<vi>, "Value"=w258:sgl)  [unwired: 1 in, 1 out]
                n136 = call "数字键盘.vi"("OldNumber"=w258) -> ("NewNumber"=w260:dbl)  [unwired: 1 in]
                n137 = property class="DigNum (严格)"(reference=w259, "Val(Sgnl)"=w260) -> ()  [unwired: 1 in, 2 out]
              }
              frame True {
              }
            }
            n138 = call "Add State to Queue.vi"("State(s) In (\"\")"=w254) -> ("States Out"=w257:string)  [unwired: 14 in]
          }
          event "大气压力": Value Change {
            n139 = event-data() -> ("NewVal"=w266:dbl)  [unwired: 1 in, 3 out]
            n140 = global read "多参数全局变量.vi" "MB session in"() -> (w267:refnum<class "MB_Master.lvclass">)
            n141 = call "纳清DO_大气压力写入.vi"("数值"=w266, "MB session in"=w267) -> ("error out"=w264:errorcluster)  [unwired: 8 in, 1 out]
            n142 = Enqueue Element At Opposite End(queue=w263, element=T1."DO" ("元素"), error in (no error)=w264) -> ()  [unwired: 1 in, 3 out]
            n143 = call "Add State to Queue.vi"("State(s) In (\"\")"=w265) -> ("States Out"=w269:string)  [unwired: 14 in]
          }
          event "滤波设定": Value Change {
            n144 = event-data() -> ()  [unwired: 1 in, 4 out]
            n145 = flat-sequence {
              frame #0 {
                n146 = global read "断电保存变量.vi" "滤波设置"() -> (w275:T4)
                n147 = local read "滤波设定"() -> (w273:dbl)
                n148 = Bundle By Name(cluster=w275, "DO"=w273) -> (w274:T4)
                n149 = global write "断电保存变量.vi" "滤波设置"(w274) -> ()
              }
              frame #1 {
                n150 = call "配置文件保存.vi"() -> ()  [unwired: 12 in]
              }
            }
            n151 = call "Add State to Queue.vi"("State(s) In (\"\")"=w270) -> ("States Out"=w272:string)  [unwired: 14 in]
          }
          event "校准启动": Value Change {
            n152 = event-data() -> ()  [unwired: 1 in, 6 out]
            n153 = global read "多参数全局变量.vi" "校准运行状态"() -> (w277:T7)
            n154 = call "Add State to Queue.vi"("State(s) In (\"\")"=w282, "State(s) At Back (\"\")"="init: all\nCal: Place standard solution\n Cal: Calibration process\nidle" ("State(s) In (\"\")")) -> ("States Out"=w281:string)  [unwired: 13 in]
            n155 = Bundle By Name(cluster=w277, "DO"=TRUE) -> (w278:T7)
            n156 = global write "多参数全局变量.vi" "校准运行状态"(w278) -> ()
          }
          event "校准停止": Value Change {
            n157 = event-data() -> ()  [unwired: 1 in, 6 out]
            n158 = call "Add State to Queue.vi"("State(s) In (\"\")"="init: all\nCal: Over\nidle" ("State(s) In (\"\")")) -> ("States Out"=w284:string)  [unwired: 14 in]
          }
          event "盐度自动获取", "盐度": Value Change {
            n159 = event-data() -> ()  [unwired: 1 in, 6 out]
            n160 = flat-sequence {
              frame #0 {
                n161 = local read "盐度"() -> (w289:sgl)
                n162 = global write "断电保存变量.vi" "盐度自动获取"("盐度自动获取") -> ()
                n163 = global write "断电保存变量.vi" "盐度补偿"(w289) -> ()
              }
              frame #1 {
                n164 = call "配置文件保存.vi"() -> ()  [unwired: 12 in]
              }
            }
            n165 = call "Add State to Queue.vi"("State(s) In (\"\")"=w288) -> ("States Out"=w287:string)  [unwired: 14 in]
          }
        }
      }
    }
  }
